vi "Set Icon.vi"(0 "VI":refnum<vi>, 5 "user-supplied text (\"\" - use VI file name)":string, 11 "error in":errorcluster) -> (4 "Error Message":string, 15 "error out":errorcluster)   [LabVIEW 2021, in "Text-Based VI Icon.lvlib"]
uses:
  Text-Based VI Icon.lvlib
  Library Icon Information.ctl
  User Visible Strings.vi
  lv_icon/Classes/Icon/Icon.lvclass
  LabVIEW Icon API.lvlib
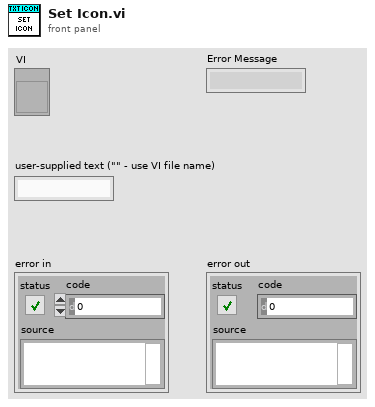
[diagram p1: front panel]
types:
  T1 = typedef "Text-Based VI Icon.lvlib/Library Icon Information.ctl" = cluster{"Library Path":path, "Number of Pixel Rows in Icon":i32, "Icon Image":picture}
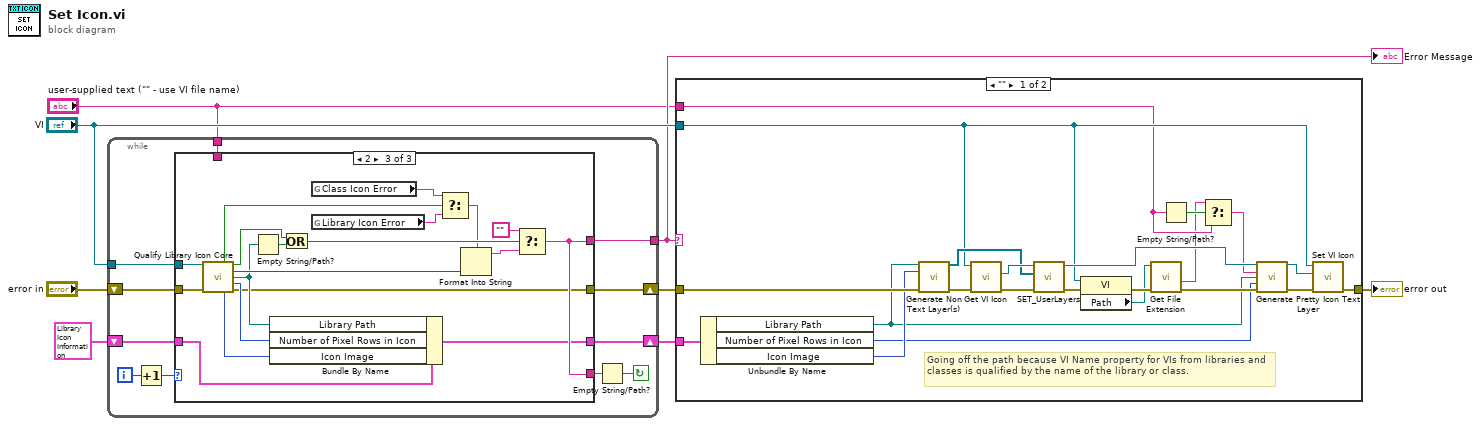
[diagram p0: block diagram]
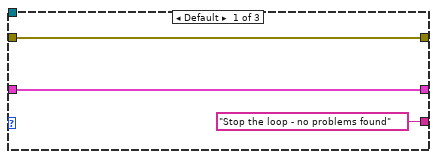
[diagram p3: hidden frame]
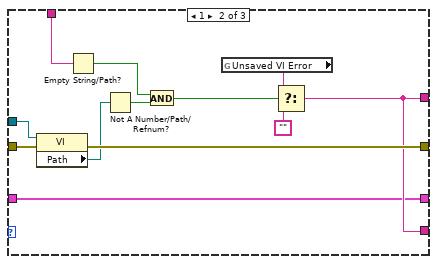
[diagram p4: hidden frame]
diagram:
  n1 = while {
    tunnel: "VI" -> [w17]
    shift-right: [w18] -> w6
    shift-left: "error in" -> [w19]
    tunnel: [w14] -> w4
    shift-right: [w10] -> w2
    shift-left: T1 {"Library Path"=path "", "Number of Pixel Rows in Icon"=0, "Icon Image"=bytes[0]} ("Library Icon Information") -> [w11]
    tunnel: "user-supplied text (\"\" - use VI file name)" -> [w9]
    i -> [w15]
    stop <- w13 continue-if-true
    n2 = Increment(x=w15) -> (x+1=w16:i32)
    n3 = case shown="2" w16 {
      tunnel: w19 -> [w22 w34 w51]
      tunnel: [w22 w33 w35] -> w18
      tunnel: w17 -> [_ w32 w52]
      tunnel: [_ w28 w53] -> w14
      tunnel: ["Stop the loop - no problems found" w28 w53] -> w12
      tunnel: w11 -> [w20 w26 w39]
      tunnel: [w20 w26 w38] -> w10
      tunnel: w9 -> [_ w25 _]
      frame Default {
      }
      frame 1 {
        n4 = property class="VI"(reference=w32, error in=w34) -> (error out=w33:errorcluster, "Path"=w31:path)  [unwired: 1 out]
        n5 = Empty String/Path?(string/path=w25) -> (empty?=w23:bool)
        n6 = Not A Number/Path/Refnum?(number/path/refnum=w31) -> (NaN/Path/Refnum?=w30:bool)
        n7 = And(x=w23, y=w30) -> (x .and. y?=w24:bool)
        n8 = global read "User Visible Strings.vi" "Unsaved VI Error"() -> (w27:string)
        n9 = Select(t=w27, s=w24, f="") -> (s? t:f=w28:string)
      }
      frame 2 {
        n10 = call "Qualify Library Icon Core.vi"("VI Reference"=w52, "error in"=w51) -> ("Class?"=w43:bool, "Good Library Icon"=w50:bool, "Maximum Number of Rows"=w45:i32, "Library Path"=w40:path, "Number of Rows in Icon"=w37:i32, "Icon Image"=w36:picture, "error out"=w35:errorcluster)  [unwired: 7 in]
        n11 = Empty String/Path?(string/path=w40) -> (empty?=w46:bool)
        n12 = Bundle By Name(cluster=w39, "Library Path"=w40, "Number of Pixel Rows in Icon"=w37, "Icon Image"=w36) -> (w38:T1)
        n13 = Or(x=w50, y=w46) -> (x .or. y?=w48:bool)
        n14 = global read "User Visible Strings.vi" "Class Icon Error"() -> (w41:string)
        n15 = global read "User Visible Strings.vi" "Library Icon Error"() -> (w42:string)
        n16 = Select(t=w41, s=w43, f=w42) -> (s? t:f=w44:string)
        n17 = Format Into String(format string=w44, w45) -> (resulting string=w47:string)  [unwired: 2 in, 1 out]
        n18 = Select(t="", s=w48, f=w47) -> (s? t:f=w53:string)
      }
    }
    n19 = Empty String/Path?(string/path=w12) -> (empty?=w13:bool)
  }
  "Error Message" <- w4
  n20 = case shown="\"\"" w4 {
    tunnel: [w75 w76] -> w8
    tunnel: w6 -> [w66 w76]
    tunnel: "VI" -> [w62 _]
    tunnel: w2 -> [w61 _]
    tunnel: "user-supplied text (\"\" - use VI file name)" -> [w56 _]
    frame "" {
      # "Going off the path because VI Name property for VIs from libraries and classes is qualified by the name of the library or class."
      n21 = Unbundle By Name(w61) -> ("Library Path"=w59:path, "Number of Pixel Rows in Icon"=w58:i32, "Icon Image"=w60:picture)
      n22 = call "Generate Non Text Layer(s).vi"("Library Path"=w59, "new picture"=w60, "error in"=w66) -> ("Layers"=w70:refnum<class "Layer.lvclass">[], "error out"=w72:errorcluster)  [unwired: 11 in]
      n23 = call "Get VI Icon.vi"("error in (no error)"=w72, "VI Refnum in"=w62) -> ("error out"=w73:errorcluster, "Icon"=w74:refnum<class "Icon.lvclass">)  [unwired: 7 in, 1 out]
      n24 = call-dynamic "SET_UserLayers.vi"("error in (no error)"=w73, "Layers"=w70, "Icon.lvclass in"=w74) -> ("error out"=w65:errorcluster, "Icon.lvclass out"=w71:refnum<class "Icon.lvclass">)  [unwired: 7 in]
      n25 = property class="VI"(reference=w62, error in=w65) -> (error out=w64:errorcluster, "Path"=w63:path)  [unwired: 1 out]
      n26 = call <vilib>:"Get File Extension.vi"("error in (no error)"=w64, "file"=w63) -> ("error out"=w69:errorcluster, "filename without extension"=w54:string)  [unwired: 5 in, 3 out]
      n27 = Empty String/Path?(string/path=w56) -> (empty?=w57:bool)
      n28 = Select(t=w54, s=w57, f=w56) -> (s? t:f=w55:string)
      n29 = call "Generate Pretty Icon Text Layer.vi"("Icon in"=w71, "VI Name"=w55, "Library Path"=w59, "Number of Rows in Icon"=w58, "error in (no error)"=w69) -> ("Icon out"=w67:refnum<class "Icon.lvclass">, "error out"=w68:errorcluster)  [unwired: 9 in]
      n30 = call "Set VI Icon.vi"("error in (no error)"=w68, "Icon"=w67, "VI Refnum in"=w62) -> ("error out"=w75:errorcluster)  [unwired: 7 in, 1 out]
    }
    frame Default {
    }
  }
  "error out" <- w8
